vi "LiveView3.vi"() -> ()   [LabVIEW 2016]
uses:
  EDSDK-Labview.llb/kEdsProperties.ctl
  EDSDK-Labview.llb/kEdsImageSrcs.ctl
  EDSDK-Labview.llb/EDS_Errors.ctl
  <vilib>/ptbypt/NI_PtbyPt.lvlib
panel:
  in  "display":bool
  out "timediff 2":i32
  out "timediff 1":i32
  out "timediff 3":i32
  out "Array":T1[](array[plugin-control])
  out "string":string
  out "uint32":u32
  in  "inPropertyID":T2=1280 items=["Unknown"=65535, "ProductName"=2, "BodyID"=3, "OwnerName"=4, "MakerName"=5, "DateTime"=6, "FirmwareVersion"=7, "BatteryLevel"=8, "CFn"=9, "SaveTo"=11, "CurrentStorage"=12, "CurrentFolder"=13, "MyMenu"=14, "BatteryQuality"=16, "HDDirectoryStructure"=32, "ImageQuality"=256, "JpegQuality"=257, "Orientation"=258, "ICCProfile"=259, "FocusInfo"=260, "DigitalExposure"=261, "WhiteBalance"=262, "ColorTemperature"=263, "WhiteBalanceShift"=264, "Contrast"=265, "ColorSaturation"=266, "ColorTone"=267, "Sharpness"=268, "ColorSpace"=269, "ToneCurve"=270, "PhotoEffect"=271, "FilterEffect"=272, "ToningEffect"=273, "ParameterSet"=274, "ColorMatrix"=275, "PictureStyle"=276, "PictureStyleDesc"=277, "ETTL2Mode"=279, "PictureStyleCaption"=512, "Linear"=768, "ClickWBPoint"=769, "WBCoeffs"=770, "GPSVersionID"=2048, "GPSLatitudeRef"=2049, "GPSLatitude"=2050, "GPSLongitudeRef"=2051, "GPSLongitude"=2052, "GPSAltitudeRef"=2053, "GPSAltitude"=2054, "GPSTimeStamp"=2055, "GPSSatellites"=2056, "GPSStatus"=2057, "GPSMapDatum"=2066, "GPSDateStamp"=2077, "AtCapture_Flag"=2147483648, "AEMode"=1024, "DriveMode"=1025, "ISOSpeed"=1026, "MeteringMode"=1027, "AFMode"=1028, "Av"=1029, "Tv"=1030, "ExposureCompensation"=1031, "FlashCompensation"=1032, "FocalLength"=1033, "AvailableShots"=1034, "Bracket"=1035, "WhiteBalanceBracket"=1036, "LensName"=1037, "AEBracket"=1038, "FEBracket"=1039, "ISOBracket"=1040, "NoiseReduction"=1041, "FlashOn"=1042, "RedEye"=1043, "FlashMode"=1044, "LensStatus"=1046, "Artist"=1048, "Copyright"=1049, "DepthOfField"=1051, "EFCompensation"=1054, "Evf_OutputDevice"=1280, "Evf_Mode"=1281, "Evf_WhiteBalance"=1282, "Evf_ColorTemperature"=1283, "Evf_DepthOfFieldPreview"=1284, "Evf_Zoom"=1287, "Evf_ZoomPosition"=1288, "Evf_FocusAid"=1289, "Evf_Histogram"=1290, "Evf_ImagePosition"=1291, "Evf_HistogramStatus"=1292, "Evf_AFMode"=1294, "Evf_CoordinateSystem"=1344, "Evf_ZoomRect"=1345]
  in  "Image Type":T3=4 items=["Grayscale (U8)", "Grayscale (I16)", "Grayscale (SGL)", "Complex (CSG)", "RGB (U32)", "HSL (U32)", "RGB (U64)", "Grayscale (U16)"]
  out "live fps":dbl format="%#_2g"
  in  "stop":bool
  out "cameras":u32
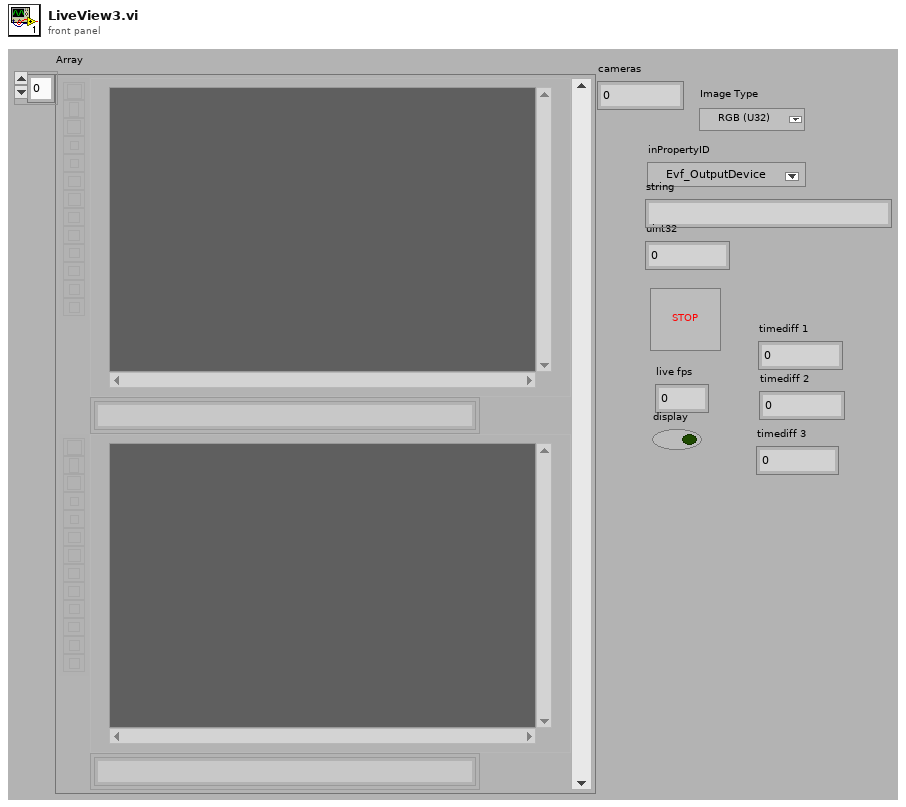
[diagram p1: front panel]
types:
  T1 = typedef "IMAQ Image.ctl" = refnum<image>
  T2 = typedef "kEdsProperties.ctl" = u32
  T3 = typedef "Image Type" = u32
  T4 = typedef "kEdsImageSrcs.ctl" = u32
  T5 = typedef "EdsImageInfo.ctl" = cluster{"width":u32, "height":u32, "# components":u32, "bit depth":u32, "rect":u32[], "reserved 1":u32, "reserved 2":u32}
  T6 = typedef "EDS_Errors.ctl" = u32
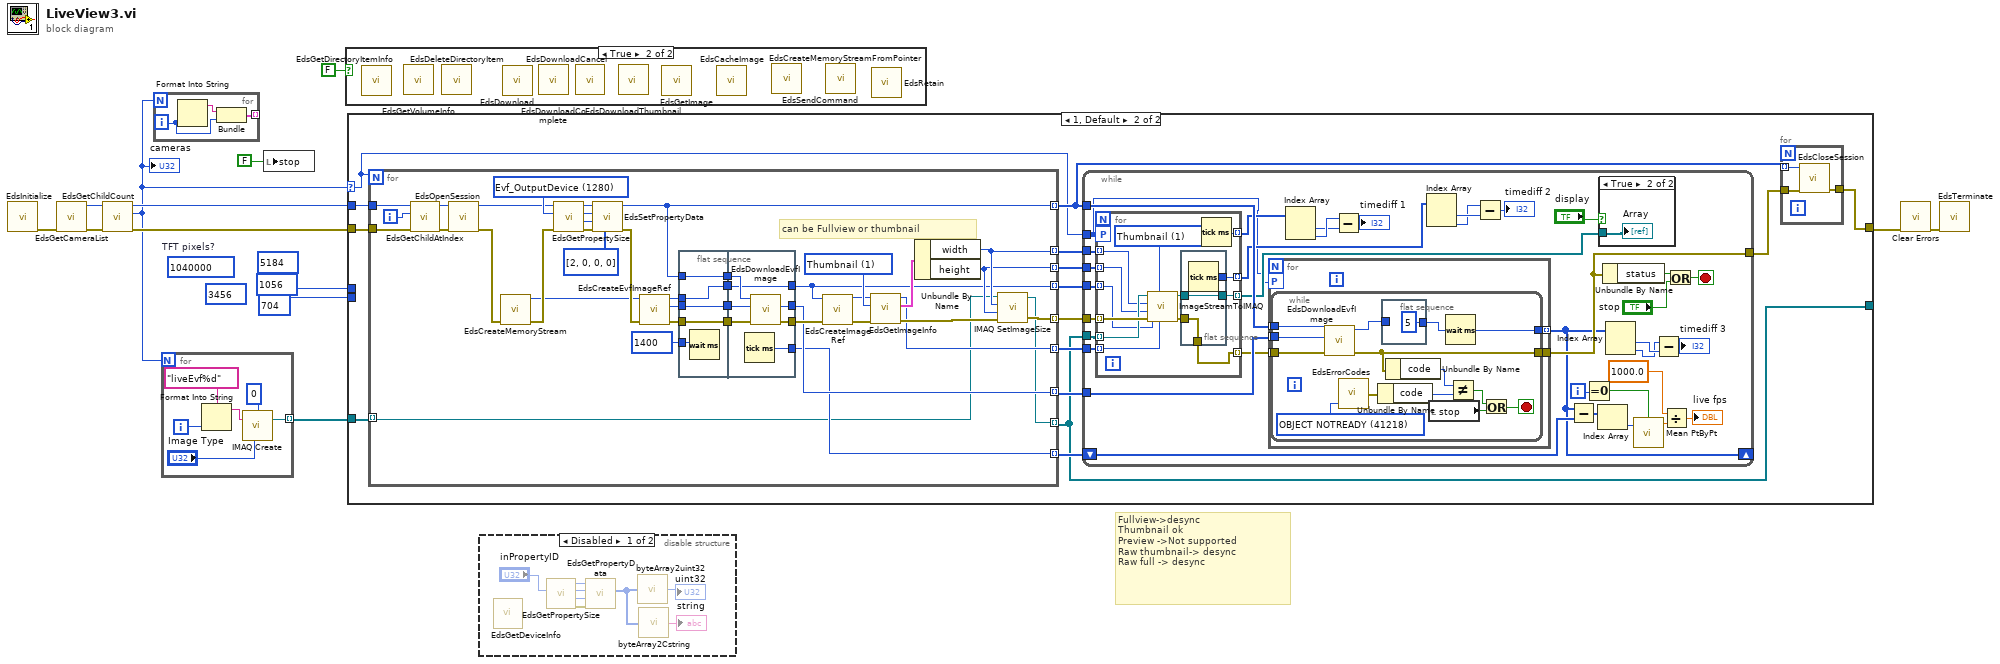
[diagram p0: block diagram]
diagram:
  (unwired) u32 1040000  # TFT pixels?
  (unwired) 3456 ("Y Resolution")
  (unwired) 5184 ("X Resolution")
  # "Fullview->desync\nThumbnail ok\nPreview ->Not supported\nRaw thumbnail-> desync\nRaw full -> desync"
  n1 = call "EdsInitialize.vi"() -> ("error out"=w13:errorcluster)  [unwired: 11 in]
  n2 = call "EdsGetCameraList.vi"("error in"=w13) -> ("error out"=w12:errorcluster, "outCameraListRef"=w10:u32)  [unwired: 9 in]
  n3 = call "EdsGetChildCount.vi"("error in"=w12, "inRef"=w10) -> ("error out"=w11:errorcluster, "count"=w2:u32, "inRef dup"=w9:u32)  [unwired: 7 in]
  "cameras" <- w2
  n4 = for {
    N: w2 -> [_]
    tunnel: [w14] -> _ mode=indexing
    i -> [w15]
    n5 = Format Into String(w15) -> (resulting string=w16:string)  [unwired: 3 in, 1 out]
    n6 = Bundle(w16, w15) -> (w14:cluster{string, i32})  [unwired: 1 in]
  }
  n7 = for {
    N: w2 -> [_]
    tunnel: [w17] -> w1 mode=indexing
    i -> [w18]
    n8 = Format Into String(format string="liveEvf%d" ("Image Name"), w18) -> (resulting string=w19:string)  [unwired: 2 in, 1 out]
    n9 = call "IMAQ Create"("Border Size"=0, "Image Name"=w19, "Image Type"="Image Type") -> ("New Image"=w17:T1)  [unwired: 2 in, 1 out]
  }
  n10 = local write "stop"(FALSE ("stop")) -> ()
  n11 = case shown="True" FALSE {
    frame False {
    }
    frame True {
      n12 = call "EdsGetDirectoryItemInfo.vi"() -> ()  [unwired: 9 in, 3 out]
      n13 = call "EdsGetVolumeInfo.vi"() -> ()  [unwired: 9 in, 3 out]
      n14 = call "EdsDeleteDirectoryItem.vi"() -> ()  [unwired: 11 in, 1 out]
      n15 = call "EdsDownload.vi"() -> ()  [unwired: 9 in, 3 out]
      n16 = call "EdsDownloadComplete.vi"() -> ()  [unwired: 11 in, 1 out]
      n17 = call "EdsDownloadCancel.vi"() -> ()  [unwired: 11 in, 1 out]
      n18 = call "EdsDownloadThumbnail.vi"() -> ()  [unwired: 9 in, 3 out]
      n19 = call "EdsGetImage.vi"() -> ()  [unwired: 10 in, 2 out]
      n20 = call "EdsCacheImage.vi"() -> ()  [unwired: 11 in, 1 out]
      n21 = call "EdsCreateMemoryStreamFromPointer.vi"() -> ()  [unwired: 10 in, 2 out]
      n22 = call "EdsSendCommand.vi"() -> ()  [unwired: 6 in, 2 out]
      n23 = call "EdsRetain.vi"() -> ()  [unwired: 9 in, 3 out]
    }
  }
  n24 = case shown="1, Default" w2 {
    selector: w2 -> [_ w25]
    tunnel: w11 -> [w24 w39]
    tunnel: w9 -> [_ w38]
    tunnel: [w24 w37] -> w8
    tunnel: [w23 w26] -> _
    tunnel: 704 ("Y Resolution") -> [_ _]
    tunnel: 1056 ("X Resolution") -> [_ _]
    tunnel: w1 -> [w23 w27]
    frame 0 {
    }
    frame 1, Default {
      n25 = for {
        N: w25 -> [_]
        tunnel: w39 -> [w78]
        tunnel: w38 -> [w77]
        tunnel: [w60] -> w36 mode=indexing
        tunnel: [w59] -> w35 mode=indexing
        tunnel: [w55] -> w33 mode=indexing
        tunnel: [w54] -> w32 mode=indexing
        tunnel: [w53] -> w31 mode=indexing
        tunnel: [w52] -> w30 mode=indexing
        tunnel: [w43] -> w26 mode=indexing
        tunnel: [w50] -> w29 mode=indexing
        tunnel: [w48] -> w28 mode=indexing
        tunnel: w27 -> [w44] mode=indexing
        i -> [w45]
        w66 = T4 1 items=["FullView", "Thumbnail", "Preview", "RAWThumbnail", "RAWFullView"] ("inImageSource")
        w69 = T2 1280 items=["Unknown"=65535, "ProductName"=2, "BodyID"=3, "OwnerName"=4, "MakerName"=5, "DateTime"=6, "FirmwareVersion"=7, "BatteryLevel"=8, "CFn"=9, "SaveTo"=11, "CurrentStorage"=12, "CurrentFolder"=13, "MyMenu"=14, "BatteryQuality"=16, "HDDirectoryStructure"=32, "ImageQuality"=256, "JpegQuality"=257, "Orientation"=258, "ICCProfile"=259, "FocusInfo"=260, "DigitalExposure"=261, "WhiteBalance"=262, "ColorTemperature"=263, "WhiteBalanceShift"=264, "Contrast"=265, "ColorSaturation"=266, "ColorTone"=267, "Sharpness"=268, "ColorSpace"=269, "ToneCurve"=270, "PhotoEffect"=271, "FilterEffect"=272, "ToningEffect"=273, "ParameterSet"=274, "ColorMatrix"=275, "PictureStyle"=276, "PictureStyleDesc"=277, "ETTL2Mode"=279, "PictureStyleCaption"=512, "Linear"=768, "ClickWBPoint"=769, "WBCoeffs"=770, "GPSVersionID"=2048, "AtCapture_Flag"=0, "AEMode"=1024, "DriveMode"=1025, "ISOSpeed"=1026, "MeteringMode"=1027, "AFMode"=1028, "Av"=1029, "Tv"=1030, "ExposureCompensation"=1031, "FlashCompensation"=1032, "FocalLength"=1033, "AvailableShots"=1034, "Bracket"=1035, "WhiteBalanceBracket"=1036, "LensName"=1037, "AEBracket"=1038, "FEBracket"=1039, "ISOBracket"=1040, "NoiseReduction"=1041, "FlashOn"=1042, "RedEye"=1043, "FlashMode"=1044, "LensStatus"=1046, "Artist"=1048, "Copyright"=1049, "DepthOfField"=1051, "EFCompensation"=1054, "Evf_OutputDevice"=1280, "Evf_Mode"=1281, "Evf_WhiteBalance"=1282, "Evf_ColorTemperature"=1283, "Evf_DepthOfFieldPreview"=1284, "Evf_Zoom"=1287, "Evf_ZoomPosition"=1288, "Evf_FocusAid"=1289, "Evf_Histogram"=1290, "Evf_ImagePosition"=1291, "Evf_HistogramStatus"=1292, "Evf_AFMode"=1294, "Evf_CoordinateSystem"=1344, "Evf_ZoomRect"=1345] ("inPropertyID")
        # "can be Fullview or thumbnail"
        n26 = call "EdsGetChildAtIndex.vi"("error in"=w78, "index"=w45, "inRef"=w77) -> ("error out"=w75:errorcluster, "outRef"=w76:u32)  [unwired: 7 in]
        n27 = call "EdsOpenSession.vi"("error in"=w75, "inCameraRef"=w76) -> ("error out"=w46:errorcluster, "inCameraRef dup"=w47:u32)  [unwired: 8 in]
        n28 = call "EdsCreateMemoryStream.vi"("error in"=w46) -> ("error out"=w62:errorcluster, "outStreamRef"=w61:u32)  [unwired: 9 in]
        n29 = call "EdsGetPropertySize.vi"("error in"=w62, "inPropertyID"=w69, "inRef"=w47) -> ("error out"=w73:errorcluster, "outSize"=w72:u32, "inPropertyID dup"=w51:T2, "inRef dup"=w74:u32)  [unwired: 4 in, 1 out]
        n30 = call "EdsSetPropertyData.vi"("inPropertyData"=u8[] [2, 0, 0, 0], "error in"=w73, "inPropertySize"=w72, "inPropertyID"=w51, "inRef"=w74) -> ("error out"=w70:errorcluster, "inRef dup"=w53:u32)  [unwired: 5 in]
        n31 = call "EdsCreateEvfImageRef.vi"("error in"=w70, "inStream"=w61) -> ("error out"=w57:errorcluster, "outEvfImage"=w67:u32, "inStream dup"=w58:u32)  [unwired: 7 in]
        n32 = flat-sequence {
          tunnel: w53 -> [w85]
          tunnel: w67 -> [w86]
          tunnel: w57 -> [w87]
          tunnel: [w87] -> w82
          tunnel: [w86] -> w81
          tunnel: [w85] -> w80
          tunnel: u32 1400 ("X Resolution") -> [w84]
          tunnel: [w83] -> w79
          tunnel: w58 -> [w83]
          tunnel: [w94] -> w56
          tunnel: w82 -> [w93]
          tunnel: w81 -> [w92]
          tunnel: w80 -> [w91]
          tunnel: [w90] -> w55
          tunnel: w79 -> [w90]
          tunnel: [w89] -> w52
          tunnel: [w88] -> w50
          frame #0 {
            n33 = Wait (ms)(milliseconds to wait=w84) -> ()  [unwired: 1 out]
          }
          frame #1 {
            n34 = Tick Count (ms)() -> (millisecond timer value=w88:u32)
            n35 = call "EdsDownloadEvfImage.vi"("error in"=w93, "inEvfImageRef"=w92, "inCameraRef"=w91) -> ("error out"=w94:errorcluster, "inEvfImageRef dup"=w89:u32)  [unwired: 6 in, 1 out]
          }
        }
        n36 = call "EdsCreateImageRef.vi"("error in"=w56, "inStreamRef"=w55) -> ("error out"=w64:errorcluster, "outImageRef"=w65:u32)  [unwired: 8 in]
        n37 = call "EdsGetImageInfo.vi"("error in"=w64, "inImageSource"=w66, "inImageRef"=w65) -> ("error out"=w49:errorcluster, "outImageInfo"=w63:T5, "inImageRef dup"=w48:u32)  [unwired: 6 in]
        n38 = Unbundle By Name(w63) -> ("width"=w60:u32, "height"=w59:u32)
        n39 = call "IMAQ SetImageSize"("error in (no error)"=w49, "Y Resolution"=w59, "X Resolution"=w60, "Image"=w44) -> ("error out"=w54:errorcluster, "Image Out"=w43:T1)  [unwired: 1 in]
      }
      n40 = while {
        tunnel: w36 -> [w114]
        tunnel: w35 -> [w113]
        tunnel: w26 -> [w116]
        tunnel: [w121] -> w34
        tunnel: w33 -> [w115]
        tunnel: w32 -> [w118]
        tunnel: w31 -> [w130]
        tunnel: w30 -> [w129]
        shift-right: [w109] -> _
        shift-left: w29 -> [w125]
        tunnel: w28 -> [w112]
        tunnel: w25 -> [w95]
        i -> [w120]
        stop <- w126 stop-if-true
        n41 = for {
          tunnel: w118 -> [w164] mode=indexing
          tunnel: [w156] -> w117 mode=indexing
          tunnel: w116 -> [w163] mode=indexing
          tunnel: w115 -> [w162] mode=indexing
          tunnel: w114 -> [w161] mode=indexing
          tunnel: w113 -> [w160] mode=indexing
          tunnel: w112 -> [w159] mode=indexing
          workers-P: w95 -> [_]
          tunnel: [w157] -> w102 mode=indexing
          tunnel: [w153] -> w96 mode=indexing
          tunnel: [w152] -> w98 mode=indexing
          w158 = T4 1 items=["FullView", "Thumbnail", "Preview", "RAWThumbnail", "RAWFullView"] ("inImageSource (Thumbnail for evf)")
          n42 = call "ImageStreamToIMAQ.vi"("inStreamRef"=w162, "inImageRef"=w159, "inImageSource (Thumbnail for evf)"=w158, "error in"=w164, "height"=w160, "width"=w161, "Image"=w163) -> ("error out"=w155:errorcluster, "Image Out"=w154:T1)  [unwired: 3 in]
          n43 = flat-sequence {
            tunnel: [w167] -> w156
            tunnel: w155 -> [w167]
            tunnel: [w166] -> w153
            tunnel: w154 -> [w166]
            tunnel: [w165] -> w152
            frame #0 {
              n44 = Tick Count (ms)() -> (millisecond timer value=w165:u32)
            }
          }
          n45 = Tick Count (ms)() -> (millisecond timer value=w157:u32)
        }
        n46 = for {
          tunnel: w130 -> [w136] mode=indexing
          tunnel: w129 -> [w135] mode=indexing
          tunnel: [w134] -> w109 mode=indexing
          tunnel: [w133] -> w121
          tunnel: w117 -> [w132] mode=indexing
          workers-P: w95 -> [_]
          n47 = while {
            tunnel: w132 -> [w150]
            tunnel: [w145] -> w133
            tunnel: w136 -> [w149]
            tunnel: w135 -> [w148]
            tunnel: [w140] -> w134
            stop <- w141 stop-if-true
            w147 = T6 41218 items=["OK"=0, "UNIMPLEMENTED"=1, "INTERNAL ERROR"=2, "MEM ALLOC FAILED"=3, "MEM FREE FAILED"=4, "OPERATION CANCELLED"=5, "INCOMPATIBLE VERSION"=6, "NOT SUPPORTED"=7, "UNEXPECTED EXCEPTION"=8, "PROTECTION VIOLATION"=9, "MISSING SUBCOMPONENT"=10, "SELECTION UNAVAILABLE"=11, "FILE IO ERROR"=32, "FILE TOO MANY OPEN"=33, "FILE NOT FOUND"=34, "FILE OPEN ERROR"=35, "FILE CLOSE ERROR"=36, "FILE SEEK ERROR"=37, "FILE TELL ERROR"=38, "FILE READ ERROR"=39, "FILE WRITE ERROR"=40, "FILE PERMISSION ERROR"=41, "FILE DISK FULL ERROR"=42, "FILE ALREADY EXISTS"=43, "FILE FORMAT UNRECOGNIZED"=44, "FILE DATA CORRUPT"=45, "FILE NAMING NA"=46, "DIR NOT FOUND"=64, "DIR IO ERROR"=65, "DIR ENTRY NOT FOUND"=66, "DIR ENTRY EXISTS"=67, "DIR NOT EMPTY"=68, "PROPERTIES UNAVAILABLE"=80, "PROPERTIES MISMATCH"=81, "PROPERTIES NOT LOADED"=83, "INVALID PARAMETER"=96, "INVALID HANDLE"=97, "INVALID POINTER"=98, "INVALID INDEX"=99, "INVALID LENGTH"=100, "INVALID FN POINTER"=101, "INVALID SORT FN"=102, "DEVICE NOT FOUND"=128, "DEVICE BUSY"=129, "DEVICE INVALID"=130, "DEVICE EMERGENCY"=131, "DEVICE MEMORY FULL"=132, "DEVICE INTERNAL ERROR"=133, "DEVICE INVALID PARAMETER"=134, "DEVICE NO DISK"=135, "DEVICE DISK ERROR"=136, "DEVICE CF GATE CHANGED"=137, "DEVICE DIAL CHANGED"=138, "DEVICE NOT INSTALLED"=139, "DEVICE STAY AWAKE"=140, "DEVICE NOT RELEASED"=141, "STREAM IO ERROR"=160, "STREAM NOT OPEN"=161, "STREAM ALREADY OPEN"=162, "STREAM OPEN ERROR"=163, "STREAM CLOSE ERROR"=164, "STREAM SEEK ERROR"=165, "STREAM TELL ERROR"=166, "STREAM READ ERROR"=167, "STREAM WRITE ERROR"=168, "STREAM PERMISSION ERROR"=169, "STREAM COULDNT BEGIN THREAD"=170, "STREAM BAD OPTIONS"=171, "STREAM END OF STREAM"=172, "COMM PORT IS IN USE"=192, "COMM DISCONNECTED"=193, "COMM DEVICE INCOMPATIBLE"=194, "COMM BUFFER FULL"=195, "COMM USB BUS ERR"=196, "USB DEVICE LOCK ERROR"=208, "USB DEVICE UNLOCK ERROR"=209, "STI UNKNOWN ERROR"=224, "STI INTERNAL ERROR"=225, "STI DEVICE CREATE ERROR"=226, "STI DEVICE RELEASE ERROR"=227, "DEVICE NOT LAUNCHED"=228, "ENUM NA"=240, "INVALID FN CALL"=241, "HANDLE NOT FOUND"=242, "INVALID ID"=243, "WAIT TIMEOUT ERROR"=244, "SESSION NOT OPEN"=8195, "INVALID TRANSACTIONID"=8196, "INCOMPLETE TRANSFER"=8199, "INVALID STRAGEID"=8200, "DEVICEPROP NOT SUPPORTED"=8202, "INVALID OBJECTFORMATCODE"=8203, "SELF TEST FAILED"=8209, "PARTIAL DELETION"=8210, "SPECIFICATION BY FORMAT UNSUPPORTED"=8212, "NO VALID OBJECTINFO"=8213, "INVALID CODE FORMAT"=8214, "UNKNOWN VENDOR CODE"=8215, "CAPTURE ALREADY TERMINATED"=8216, "INVALID PARENTOBJECT"=8218, "INVALID DEVICEPROP FORMAT"=8219, "INVALID DEVICEPROP VALUE"=8220, "SESSION ALREADY OPEN"=8222, "TRANSACTION CANCELLED"=8223, "SPECIFICATION OF DESTINATION UNSUPPORTED"=8224, "UNKNOWN COMMAND"=40961, "OPERATION REFUSED"=40965, "LENS COVER CLOSE"=40966, "LOW BATTERY"=41217, "OBJECT NOTREADY"=41218, "TAKE PICTURE AF NG"=36097, "TAKE PICTURE RESERVED"=36098, "TAKE PICTURE MIRROR UP NG"=36099, "TAKE PICTURE SENSOR CLEANING NG"=36100, "TAKE PICTURE SILENCE NG"=36101, "TAKE PICTURE NO CARD NG"=36102, "TAKE PICTURE CARD NG"=36103, "TAKE PICTURE CARD PROTECT NG"=36104, "TAKE PICTURE MOVIE CROP NG"=36105, "TAKE PICTURE STROBO CHARGE NG"=36106, "LAST GENERIC ERROR PLUS ONE"=245] ("EDS_Error code")
            n48 = call "EdsDownloadEvfImage.vi"("error in"=w150, "inEvfImageRef"=w148, "inCameraRef"=w149) -> ("error out"=w145:errorcluster, "inCameraRef dup"=w137:u32)  [unwired: 6 in, 1 out]
            n49 = call "EdsErrorCodes.vi"("EDS_Error code"=w147) -> ("error out"=w146:errorcluster)  [unwired: 4 in]
            n50 = Unbundle By Name(w146) -> ("code"=w138:i32)
            n51 = flat-sequence {
              tunnel: [u32 5 ("milliseconds to wait")] -> w144
              tunnel: w137 -> [_]
              frame #0 {
              }
            }
            n52 = Unbundle By Name(w145) -> ("code"=w139:i32)
            n53 = local read "stop"() -> (w143:bool)
            n54 = Wait (ms)(milliseconds to wait=w144) -> (millisecond timer value=w140:u32)
            n55 = Not Equal?(x=w139, y=w138) -> (x != y?=w142:bool)
            n56 = Or(x=w142, y=w143) -> (x .or. y?=w141:bool)
          }
        }
        n57 = Index Array(array=w102) -> (element #1=w104:u32, element #2=w105:u32)  [unwired: 2 in]
        n58 = Subtract(x=w105, y=w104) -> (x-y=→"timediff 1":u32)
        n59 = Index Array(array=w98) -> (element #1=w100:u32, element #2=w99:u32)  [unwired: 2 in]
        n60 = Subtract(x=w99, y=w100) -> (x-y=→"timediff 2":u32)
        n61 = Subtract(x=w109, y=w125) -> (x-y=w111:u32[])
        n62 = Equal To 0?(x=w120) -> (x = 0?=w119:bool)
        n63 = Index Array(array=w111) -> (element=w110:u32)  [unwired: 1 in]
        n64 = case shown="True" "display" {
          tunnel: w96 -> [_ w131]
          frame False {
          }
          frame True {
            "Array" <- w131
          }
        }
        n65 = Unbundle By Name(w121) -> ("status"=w128:bool)
        n66 = Index Array(array=w109) -> (element #1=w107:u32, element #2=w106:u32)  [unwired: 2 in]
        n67 = call <vilib>:"Mean PtByPt.vi"("x"=w110, "initialize"=w119) -> ("mean"=w124:dbl)  [unwired: 2 in, 1 out]
        n68 = Subtract(x=w106, y=w107) -> (x-y=→"timediff 3":u32)
        n69 = Divide(x=1000.0, y=w124) -> (x/y=→"live fps":dbl)
        n70 = Or(x=w128, y="stop") -> (x .or. y?=w126:bool)
      }
      n71 = for {
        tunnel: [w42] -> w37
        tunnel: w34 -> [w41]
        tunnel: w31 -> [w40] mode=indexing
        n72 = call "EdsCloseSession.vi"("error in"=w41, "inCameraRef"=w40) -> ("error out"=w42:errorcluster)  [unwired: 8 in, 1 out]
      }
    }
  }
  n73 = disable-structure shown="Disabled" {
    frame Disabled {
      n74 = call "EdsGetDeviceInfo.vi"() -> ()  [unwired: 9 in, 3 out]
      n75 = call "EdsGetPropertySize.vi"("inPropertyID"="inPropertyID") -> ("error out"=w172:errorcluster, "outSize"=w174:u32, "inPropertyID dup"=w168:T2, "inRef dup"=w175:u32)  [unwired: 6 in, 1 out]
      n76 = call "EdsGetPropertyData.vi"("error in"=w172, "inPropertySize"=w174, "inPropertyID"=w168, "inRef"=w175) -> ("outPropertyData"=w169:u8[])  [unwired: 5 in, 2 out]
      n77 = call "byteArray2uint32.vi"("byteArray"=w169) -> ("uint32"=→"uint32":u32)
      n78 = call "byteArray2Cstring.vi"("byteArray"=w169) -> ("string"=→"string":string)
    }
    frame Enabled {
    }
  }
  n79 = call <vilib>:"Clear Errors.vi"("error in (no error)"=w8) -> ("error out"=w7:errorcluster)  [unwired: 5 in, 1 out]
  n80 = call "EdsTerminate.vi"("error in"=w7) -> ()  [unwired: 10 in, 1 out]
